vi "测量系统1042.vi"() -> ()   [LabVIEW 2012]
uses:
  <vilib>/Instr/_visa.llb/VISA Configure Serial Port (Instr).vi
panel:
  out "输出变量":dbl
  out "数值":i32
  in  "Time Target (s)":dbl=1.0 caption="目标时间(s)"
  in  "停止":bool
  in  "元素 5":i32
  in  "元素 4":i32
  in  "元素 3":i32
  in  "元素 2":i32
  in  "元素":i32
  out "当前湿度值":dbl(knob) scale=0.0..100.0
  out "当前温度值":dbl(knob) scale=0.0..100.0
  in  "串口号：":refnum<visa-resource-name>
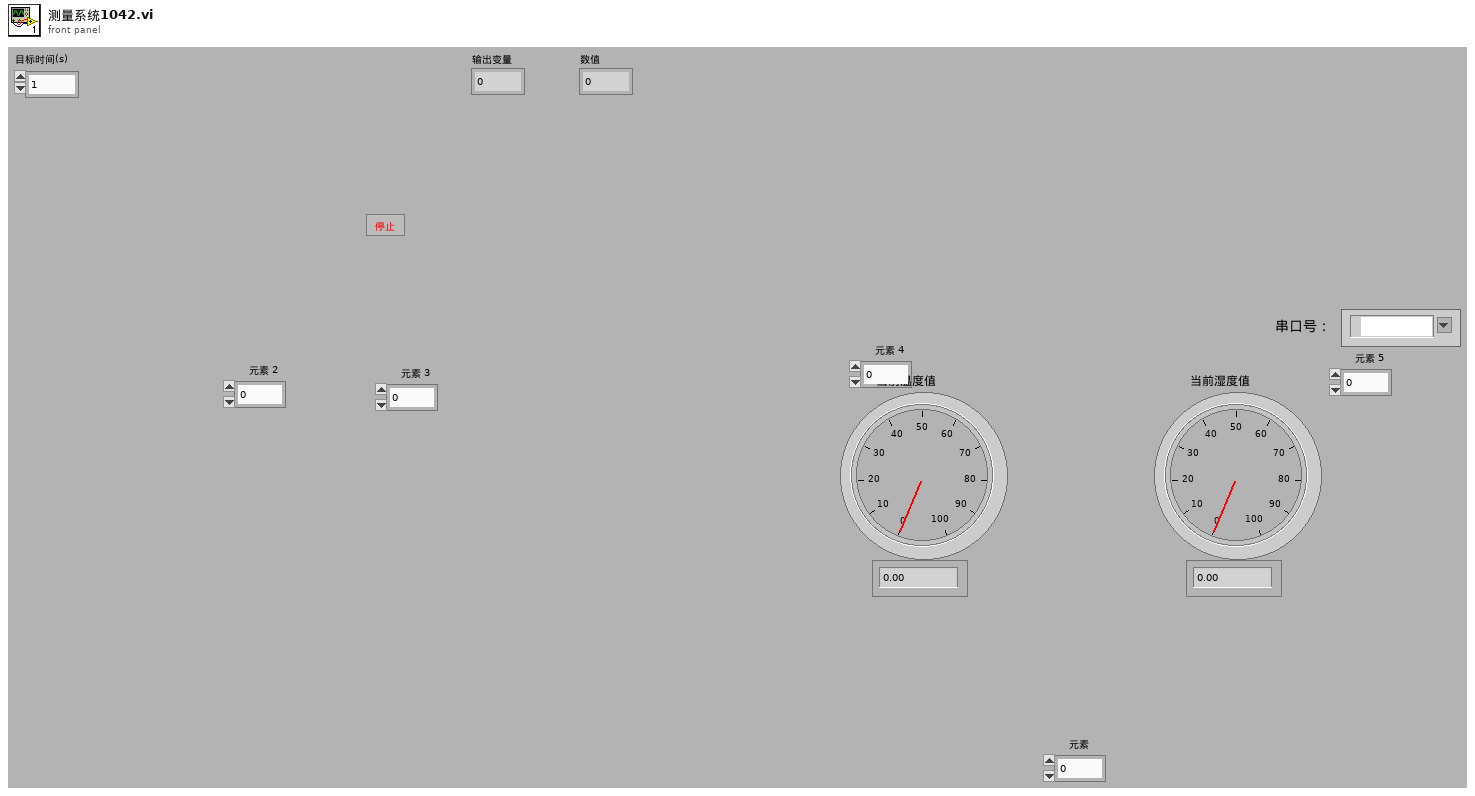
[diagram p1: front panel]
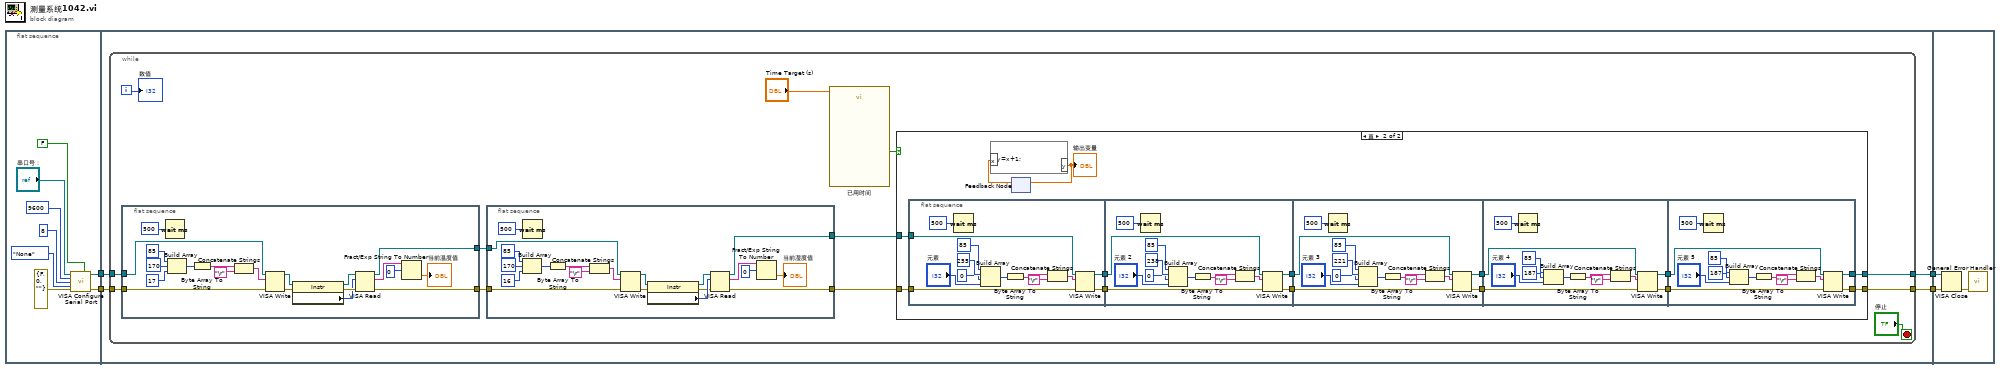
[diagram p0: block diagram]
diagram:
  n1 = flat-sequence {
    tunnel: [w7] -> w4
    tunnel: [w6] -> w3
    tunnel: w4 -> [w15]
    tunnel: w3 -> [w16]
    tunnel: [w13] -> w2
    tunnel: [w14] -> w1
    tunnel: w2 -> [w150]
    tunnel: w1 -> [w148]
    frame #0 {
      n2 = call-poly "VISA Configure Serial Port"("VISA resource name"="串口号：", "Enable Termination\nChar (T)"=FALSE ("Enable Termination\nChar (T)"), "baud rate (9600)"=u32 9600, "data bits (8)"=u16 8, "parity (0:none)"=enum16{"None", "Odd", "Even", "Mark", "Space"}."None", "error in (no error)"=errorcluster {"status"=FALSE, "code"=0, "source"=""}) -> ("VISA resource name out"=w7:refnum<visa-resource-name>, "error out"=w6:errorcluster)  [unwired: 1 in, 7 out]
    }
    frame #1 {
      n3 = while {
        tunnel: w16 -> [w28]
        tunnel: w15 -> [w27]
        tunnel: [w24] -> w14
        tunnel: [w23] -> w13
        i -> [w18]
        stop <- "停止" stop-if-true
        n4 = flat-sequence {
          tunnel: w28 -> [w147]
          tunnel: [w129] -> w22
          tunnel: [w130] -> w21
          tunnel: w27 -> [w128]
          frame #0 {
            n5 = Wait (ms)(milliseconds to wait=u32 500 ("等待时间（毫秒）")) -> ()  [unwired: 1 out]
            n6 = Build Array(85, 170, 17) -> (w145:i32[])
            n7 = Byte Array To String(unsigned byte array=w145) -> (string=w140:string)
            n8 = Concatenate Strings(w140, "\r") -> (w141:string)
            n9 = VISA Write(VISA resource name=w128, write buffer=w141, error in (no error)=w147) -> (VISA resource name out=w136:refnum<visa-resource-name>, error out=w135:errorcluster)  [unwired: 1 out]
            n10 = property class="Instr"(reference=w136, error in=w135) -> (reference out=w134:refnum<visa-resource-name>, error out=w133:errorcluster, "Serial Settings:Number of Bytes at Serial Port"=w132:u32)
            n11 = VISA Read(VISA resource name=w134, byte count=w132, error in (no error)=w133) -> (VISA resource name out=w129:refnum<visa-resource-name>, read buffer=w138:string, error out=w130:errorcluster)  [unwired: 1 out]
            n12 = Fract/Exp String To Number(string=w138, offset=0 ("偏移量")) -> (number=→"当前温度值":dbl)  [unwired: 2 in, 1 out]
          }
        }
        n13 = flat-sequence {
          tunnel: [w108] -> w26
          tunnel: w22 -> [w111]
          tunnel: [w110] -> w25
          tunnel: w21 -> [w109]
          frame #0 {
            n14 = Build Array(85, 170, 16) -> (w113:i32[])
            n15 = Wait (ms)(milliseconds to wait=u32 500 ("等待时间（毫秒）")) -> ()  [unwired: 1 out]
            n16 = Byte Array To String(unsigned byte array=w113) -> (string=w118:string)
            n17 = Concatenate Strings(w118, "\r") -> (w117:string)
            n18 = VISA Write(VISA resource name=w111, write buffer=w117, error in (no error)=w109) -> (VISA resource name out=w122:refnum<visa-resource-name>, error out=w123:errorcluster)  [unwired: 1 out]
            n19 = property class="Instr"(reference=w122, error in=w123) -> (reference out=w124:refnum<visa-resource-name>, error out=w125:errorcluster, "Serial Settings:Number of Bytes at Serial Port"=w126:u32)
            n20 = VISA Read(VISA resource name=w124, byte count=w126, error in (no error)=w125) -> (VISA resource name out=w108:refnum<visa-resource-name>, read buffer=w120:string, error out=w110:errorcluster)  [unwired: 1 out]
            n21 = Fract/Exp String To Number(string=w120, offset=0 ("偏移量")) -> (number=→"当前湿度值":dbl)  [unwired: 2 in, 1 out]
          }
        }
        n22 = call "已用时间"("Time Target (s)"="Time Target (s)") -> ("Time has Elapsed"=w17:bool)  [unwired: 11 in, 7 out]
        n23 = case shown="真" w17 {
          tunnel: w26 -> [w29 w36]
          tunnel: w25 -> [w30 w35]
          tunnel: [w29 w34] -> w24
          tunnel: [w30 w33] -> w23
          frame False {
          }
          frame True {
            n24 = flat-sequence {
              tunnel: w36 -> [w47]
              tunnel: w35 -> [w45]
              tunnel: [w50] -> w44
              tunnel: [w46] -> w43
              tunnel: w44 -> [w61]
              tunnel: w43 -> [w60]
              tunnel: [w59] -> w42
              tunnel: [w58] -> w41
              tunnel: w42 -> [w76]
              tunnel: w41 -> [w75]
              tunnel: [w74] -> w40
              tunnel: [w73] -> w39
              tunnel: w40 -> [w88]
              tunnel: w39 -> [w87]
              tunnel: [w85] -> w38
              tunnel: [w86] -> w37
              tunnel: w38 -> [w100]
              tunnel: w37 -> [w99]
              tunnel: [w98] -> w34
              tunnel: [w97] -> w33
              frame #0 {
                n25 = Wait (ms)(milliseconds to wait=u32 500 ("等待时间（毫秒）")) -> ()  [unwired: 1 out]
                n26 = Build Array(85, 255, 0 ("元素"), "元素") -> (w52:i32[])
                n27 = Byte Array To String(unsigned byte array=w52) -> (string=w57:string)
                n28 = Concatenate Strings(w57, "\r") -> (w56:string)
                n29 = VISA Write(VISA resource name=w47, write buffer=w56, error in (no error)=w45) -> (VISA resource name out=w50:refnum<visa-resource-name>, error out=w46:errorcluster)  [unwired: 1 out]
              }
              frame #1 {
                n30 = Wait (ms)(milliseconds to wait=u32 500 ("等待时间（毫秒）")) -> ()  [unwired: 1 out]
                n31 = Build Array(85, 238, 0 ("元素"), "元素 2") -> (w65:i32[])
                n32 = Byte Array To String(unsigned byte array=w65) -> (string=w70:string)
                n33 = Concatenate Strings(w70, "\r") -> (w69:string)
                n34 = VISA Write(VISA resource name=w61, write buffer=w69, error in (no error)=w60) -> (VISA resource name out=w59:refnum<visa-resource-name>, error out=w58:errorcluster)  [unwired: 1 out]
              }
              frame #2 {
                n35 = Wait (ms)(milliseconds to wait=u32 500 ("等待时间（毫秒）")) -> ()  [unwired: 1 out]
                n36 = Build Array(85, 221, 0 ("元素"), "元素 3") -> (w78:i32[])
                n37 = Byte Array To String(unsigned byte array=w78) -> (string=w83:string)
                n38 = Concatenate Strings(w83, "\r") -> (w82:string)
                n39 = VISA Write(VISA resource name=w76, write buffer=w82, error in (no error)=w75) -> (VISA resource name out=w73:refnum<visa-resource-name>, error out=w74:errorcluster)  [unwired: 1 out]
              }
              frame #3 {
                n40 = Wait (ms)(milliseconds to wait=u32 500 ("等待时间（毫秒）")) -> ()  [unwired: 1 out]
                n41 = Build Array(85, 187, "元素 4") -> (w90:i32[])
                n42 = Byte Array To String(unsigned byte array=w90) -> (string=w95:string)
                n43 = Concatenate Strings(w95, "\r") -> (w94:string)
                n44 = VISA Write(VISA resource name=w87, write buffer=w94, error in (no error)=w88) -> (VISA resource name out=w86:refnum<visa-resource-name>, error out=w85:errorcluster)  [unwired: 1 out]
              }
              frame #4 {
                n45 = Wait (ms)(milliseconds to wait=u32 500 ("等待时间（毫秒）")) -> ()  [unwired: 1 out]
                n46 = Build Array(85, 187, "元素 5") -> (w102:i32[])
                n47 = Byte Array To String(unsigned byte array=w102) -> (string=w107:string)
                n48 = Concatenate Strings(w107, "\r") -> (w106:string)
                n49 = VISA Write(VISA resource name=w99, write buffer=w106, error in (no error)=w100) -> (VISA resource name out=w98:refnum<visa-resource-name>, error out=w97:errorcluster)  [unwired: 1 out]
              }
            }
            n50 = feedback #1() -> (w32:dbl)  [unwired: 1 in]
            n51 = formula code="y=x+1;"("x"=w32) -> ("y"=w31:dbl)
            "输出变量" <- w31
            n52 = feedback-in #1(w31) -> ()
          }
        }
        "数值" <- w18
      }
    }
    frame #2 {
      n53 = VISA Close(VISA resource name=w148, error in (no error)=w150) -> (error out=w149:errorcluster)
      n54 = call <vilib>:"General Error Handler.vi"("error in (no error)"=w149) -> ()  [unwired: 10 in, 5 out]
    }
  }
